vi "Add ROI Offset ImgDataAvg.vi"(4 "Region of Interest":i32[](array[numeric])=[-1, -1, 32000, 32000], 5 "ImgData Avg In":T1={"Centroid Avg"={"X"=378.25015, "Y"=293.73102}, "Max Intensity Avg"=207.3, "Radius Avg"={"Rx"=378.25015, "Ry"=293.73102}} caption="Data Average" {"Centroid Avg"."X" format="%#_5g"; "Centroid Avg"."Y" format="%#_5g"; "Max Intensity Avg" format="%#_4g"; "Radius Avg"."Rx" format="%#_5g"; "Radius Avg"."Ry" format="%#_5g"}) -> (2 "ImgData Avg Out":T1={"Centroid Avg"={"X"=378.25015, "Y"=293.73102}, "Max Intensity Avg"=207.3, "Radius Avg"={"Rx"=378.25015, "Ry"=293.73102}} caption="Data Average" {"Centroid Avg"."X" format="%#_5g"; "Centroid Avg"."Y" format="%#_5g"; "Max Intensity Avg" format="%#_4g"; "Radius Avg"."Rx" format="%#_5g"; "Radius Avg"."Ry" format="%#_5g"})   [LabVIEW 2013]
panel:
  # "Int"
  # "Int"
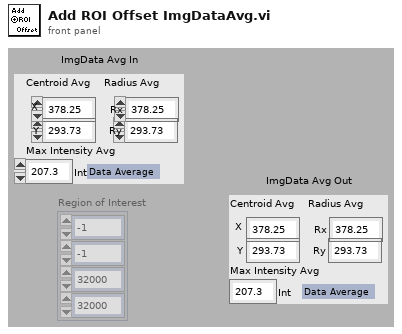
[diagram p1: front panel]
types:
  T1 = cluster{"Centroid Avg":cluster{"X":sgl, "Y":sgl}, "Max Intensity Avg":sgl, "Radius Avg":cluster{"Rx":sgl, "Ry":sgl}}
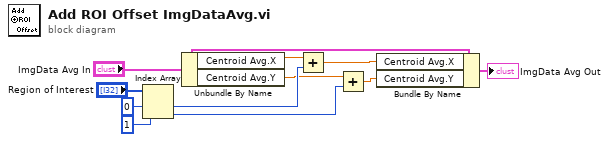
[diagram p0: block diagram]
diagram:
  n1 = Index Array(array="Region of Interest", index #1=0 ("index"), index #2=1 ("index")) -> (element #1=w8:i32, element #2=w7:i32)
  n2 = Unbundle By Name("ImgData Avg In") -> ("Centroid Avg.X"=w4:sgl, "Centroid Avg.Y"=w6:sgl)
  n3 = Add(x=w4, y=w8) -> (x+y=w5:sgl)
  n4 = Add(x=w6, y=w7) -> (x+y=w3:sgl)
  n5 = Bundle By Name(cluster="ImgData Avg In", "Centroid Avg.X"=w5, "Centroid Avg.Y"=w3) -> (→"ImgData Avg Out":T1)
